vi "Read Message to Log.vi"(8 "error in (no error)":errorcluster, 11 "MessageLoggerMessage.lvclass in":refnum<class "MessageLoggerMessage.lvclass">) -> (0 "error out":errorcluster, 1 "millisecond timer":u32, 2 "call chain":string[](array[string]), 3 "Messenging.lvlib:Interprocess Message":refnum<class "MSG.lvclass">)   [LabVIEW 2011, in "Messenging.lvlib" / "MessageLoggerMessage.lvclass"]
uses:
  MessageLoggerMessage.lvclass
  Interprocess Messenger/TextVarientMessage/MSG.lvclass
  MessageLoggerMessage.lvclass/MessageLoggerMessage.ctl
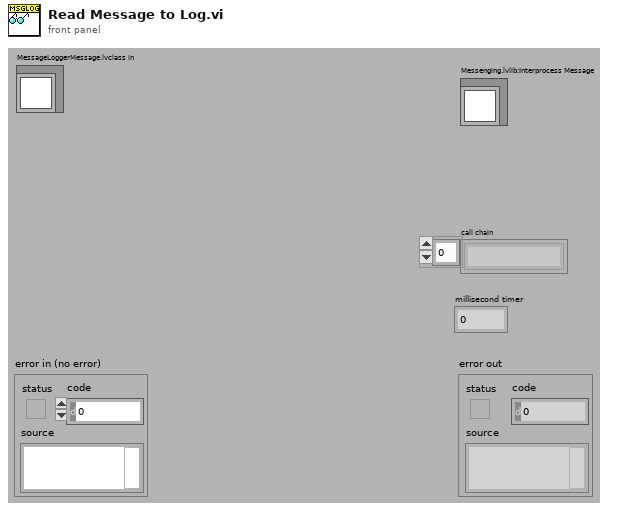
[diagram p1: front panel]
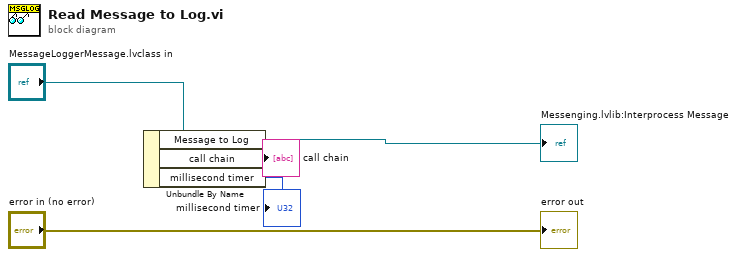
[diagram p0: block diagram]
diagram:
  n1 = Unbundle By Name("MessageLoggerMessage.lvclass in") -> ("Message to Log"=→"Messenging.lvlib:Interprocess Message":refnum<class "MSG.lvclass">, "call chain"=→"call chain":string[], "millisecond timer"=→"millisecond timer":u32)
  "error out" <- "error in (no error)"
